vi "Merit factor GUI.vi"(8 "error in (no error)":errorcluster, 11 "DAQOrcaFlash in":refnum<class "DAQOrcaFlash.lvclass">) -> (0 "error out":errorcluster, 3 "DAQOrcaFlash out":refnum<class "DAQOrcaFlash.lvclass">)   [LabVIEW 2012, in "DAQOrcaFlash.lvclass"]
uses:
  DAQOrcaFlash.lvclass
  <vilib>/Distrio/Murmex/Murmex/Murmex.lvclass
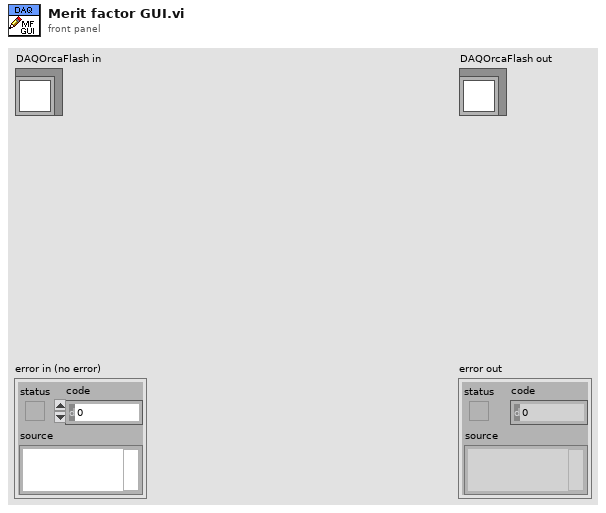
[diagram p1: front panel]
types:
  T1 = enum8{"Enabled", "Disabled", "Disabled and Grayed Out"}
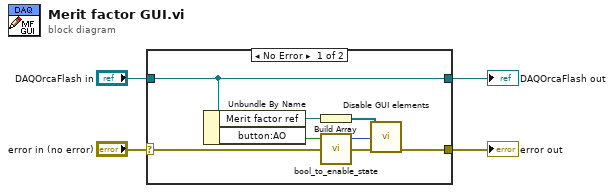
[diagram p0: block diagram]
diagram:
  n1 = case shown="No Error" "error in (no error)" {
    selector: "error in (no error)" -> [w6 w13]
    tunnel: [w5 w13] -> w3
    tunnel: [w11 w12] -> w1
    tunnel: "DAQOrcaFlash in" -> [w11 w12]
    frame No Error {
      n2 = Unbundle By Name(w11) -> ("Merit factor ref"=w10:refnum<vi>, "button:AO"=w9:bool)
      n3 = Build Array(w10) -> (w8:refnum<vi>[])
      n4 = call "bool_to_enable_state.vi"("boolean in"=w9) -> ("enabled status out"=w7:T1)  [unwired: 4 in]
      n5 = call <vilib>:"Disable GUI elements.vi"("error in (no error)"=w6, "enabled state"=w7, "control refs"=w8) -> ("error out"=w5:errorcluster)  [unwired: 8 in]
    }
    frame Error {
    }
  }
  "error out" <- w3
  "DAQOrcaFlash out" <- w1
